vi "Write Valves Ratio.vi"(8 "error in (no error)":errorcluster, 10 "Valves ratios":dbl[](array[numeric]), 11 "FPGA VI Reference In":refnum<k20>) -> (0 "error out":errorcluster, 3 "FPGA VI Reference Out":refnum<k20>)   [LabVIEW 2018, in "RT-FPGA Interface API.lvlib"]
uses:
  RT-FPGA Interface API.lvlib
  <vilib>/rvi/interface/nirviReadWriteControl/nirviReadWriteControl.xnode
  NiFpgaLv.dll
  <vilib>/Utility/error.llb/Error Cluster From Error Code.vi
  <vilib>/rvi/interface/Simulation/niFpgaSimulationCallBeginRW.vi
  <vilib>/rvi/errors/niLvFpgaAdjustHostInterfaceError.vi
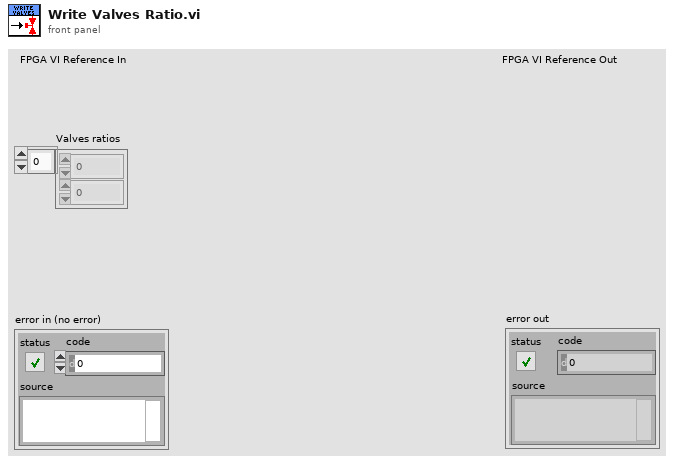
[diagram p1: front panel]
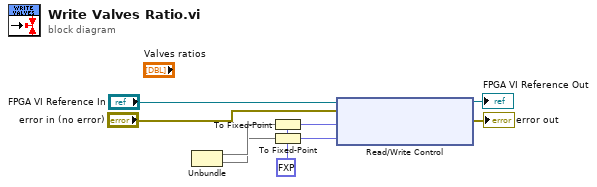
[diagram p0: block diagram]
diagram:
  w6 = fxp<+/-,20,5> 0.0 ("Bomba 1")
  n1 = Unbundle() -> (w1:cluster{"Pump 2":dbl}, w3, w2)
  n2 = To Fixed-Point(fixed-point type=w6, number=w3) -> (fixed-point=w8:fxp<+/-,20,5>)
  n3 = To Fixed-Point(fixed-point type=w6, number=w2) -> (fixed-point=w7:fxp<+/-,20,5>)
  n4 = xnode "Read/Write Control"("FPGA VI Reference In"="FPGA VI Reference In", "error in"="error in (no error)", "Valvula proporcional 1"=w8, "Valvula proporcional 2"=w7) -> ("FPGA VI Reference Out"=→"FPGA VI Reference Out":refnum<k20>, "error out"=→"error out":errorcluster)
